vi "IO通讯.vi"(6 "baud rate (9600)":u32=9600 caption="波特率(9600)", 7 "VISA resource name":refnum<visa-resource-name> caption="VISA资源名称", 8 "错误输入（无错误）":errorcluster, 9 "操作":T1(ring), 10 "WRITE AND READ":string, 11 "WRITE":string) -> (0 "错误输出":errorcluster, 3 "READ":string)   [LabVIEW 2018, in "qingshan.lvlib"]
uses:
  qingshan/qingshan.lvlib
  <vilib>/Instr/_visa.llb/VISA Configure Serial Port (Instr).vi
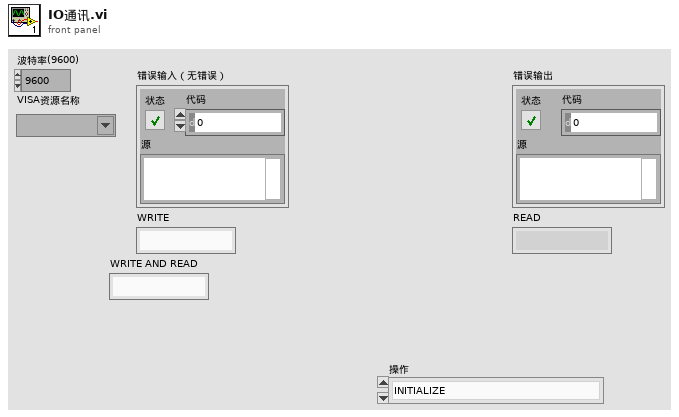
[diagram p1: front panel]
types:
  T1 = enum16{"INITIALIZE", "OPEN", "WRITE", "READ", "WRITE   AND  READ", "CLOSE", ""}
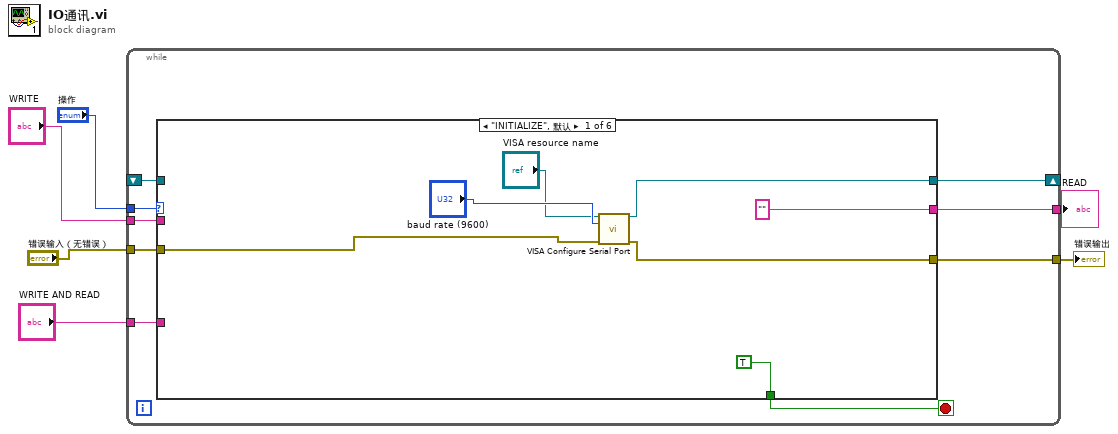
[diagram p0: block diagram]
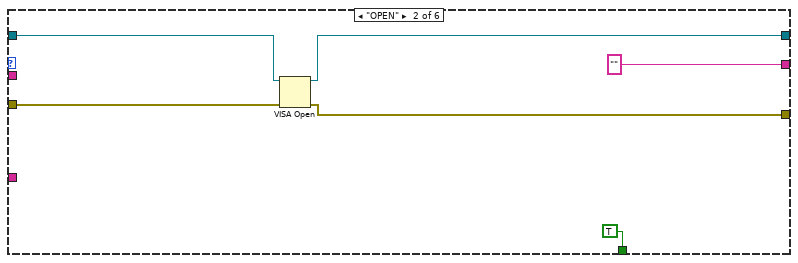
[diagram p2: hidden frame]
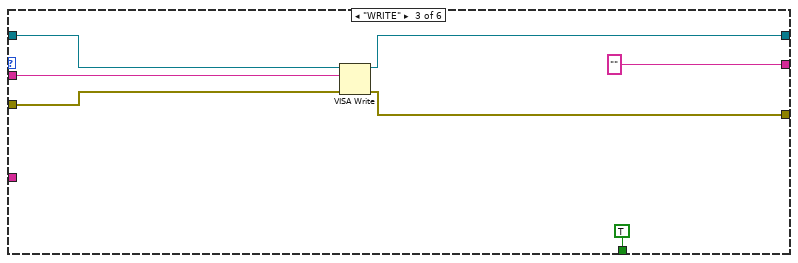
[diagram p3: hidden frame]
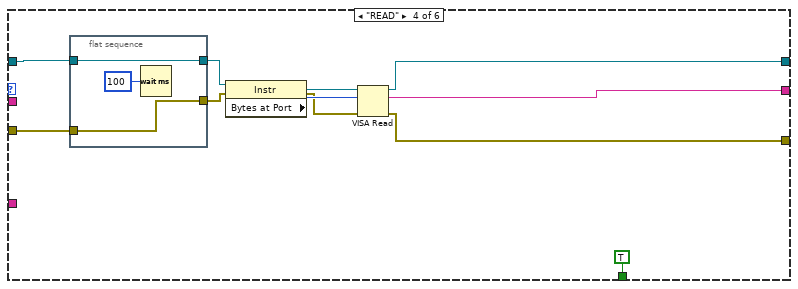
[diagram p4: hidden frame]
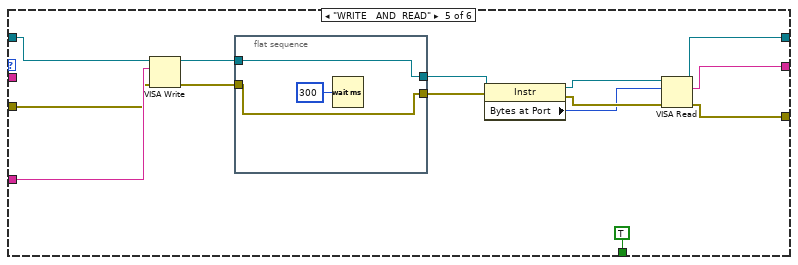
[diagram p5: hidden frame]
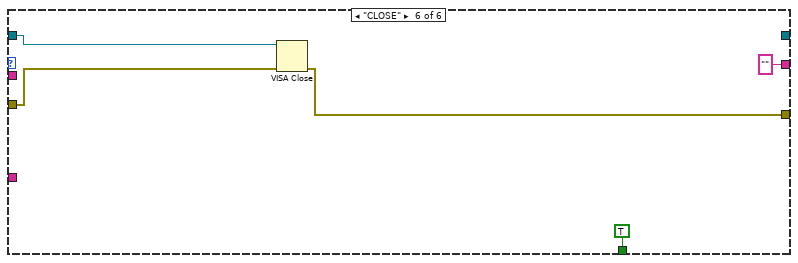
[diagram p6: hidden frame]
diagram:
  n1 = while {
    tunnel: "操作" -> [w15]
    shift-right: [w14] -> _
    shift-left: _ -> [w12]
    tunnel: "错误输入（无错误）" -> [w11]
    tunnel: [w10] -> w4
    tunnel: "WRITE" -> [w9]
    tunnel: [w8] -> w2
    tunnel: "WRITE AND READ" -> [w7]
    stop <- w13 stop-if-true
    n2 = case shown="\"INITIALIZE\", 默认" w15 {
      tunnel: [w22 w27 w34 w44 w52 _] -> w14
      tunnel: [TRUE TRUE TRUE TRUE TRUE TRUE] -> w13
      tunnel: w12 -> [_ w28 w35 w40 w62 w71]
      tunnel: w11 -> [w19 w25 w32 w38 w61 w70]
      tunnel: [w20 w24 w31 w43 w51 w69] -> w10
      tunnel: w9 -> [_ _ w33 _ _ _]
      tunnel: ["" ("read buffer") "" ("read buffer") "" ("read buffer") w42 w53 "" ("read buffer")] -> w8
      tunnel: w7 -> [_ _ _ _ w63 _]
      frame "INITIALIZE", Default {
        n3 = call-poly "VISA Configure Serial Port"("VISA resource name"="VISA resource name", "baud rate (9600)"="baud rate (9600)", "error in (no error)"=w19) -> ("VISA resource name out"=w22:refnum<visa-resource-name>, "error out"=w20:errorcluster)  [unwired: 11 in]
      }
      frame "OPEN" {
        n4 = VISA Open(error in (no error)=w25, VISA resource name=w28) -> (VISA resource name=w27:refnum<visa-resource-name>, error out=w24:errorcluster)  [unwired: 3 in]
      }
      frame "WRITE" {
        n5 = VISA Write(VISA resource name=w35, write buffer=w33, error in (no error)=w32) -> (VISA resource name out=w34:refnum<visa-resource-name>, error out=w31:errorcluster)  [unwired: 1 out]
      }
      frame "READ" {
        n6 = flat-sequence {
          tunnel: [w48] -> w41
          tunnel: w40 -> [w48]
          tunnel: [w47] -> w39
          tunnel: w38 -> [w47]
          frame #0 {
            n7 = Wait (ms)(milliseconds to wait=u32 100 ("等待时间（毫秒）")) -> ()  [unwired: 1 out]
          }
        }
        n8 = property class="Instr"(reference=w41, error in=w39) -> (reference out=w46:refnum<visa-resource-name>, error out=w37:errorcluster, "Bytes at Port"=w45:u32)
        n9 = VISA Read(VISA resource name=w46, byte count=w45, error in (no error)=w37) -> (VISA resource name out=w44:refnum<visa-resource-name>, read buffer=w42:string, error out=w43:errorcluster)  [unwired: 1 out]
      }
      frame "WRITE   AND  READ" {
        n10 = VISA Write(VISA resource name=w62, write buffer=w63, error in (no error)=w61) -> (VISA resource name out=w59:refnum<visa-resource-name>, error out=w57:errorcluster)  [unwired: 1 out]
        n11 = flat-sequence {
          tunnel: [w65] -> w60
          tunnel: w59 -> [w65]
          tunnel: [w64] -> w58
          tunnel: w57 -> [w64]
          frame #0 {
            n12 = Wait (ms)(milliseconds to wait=u32 300 ("等待时间（毫秒）")) -> ()  [unwired: 1 out]
          }
        }
        n13 = property class="Instr"(reference=w60, error in=w58) -> (reference out=w56:refnum<visa-resource-name>, error out=w55:errorcluster, "Bytes at Port"=w54:u32)
        n14 = VISA Read(VISA resource name=w56, byte count=w54, error in (no error)=w55) -> (VISA resource name out=w52:refnum<visa-resource-name>, read buffer=w53:string, error out=w51:errorcluster)  [unwired: 1 out]
      }
      frame "CLOSE" {
        n15 = VISA Close ("VISA关闭")(VISA resource name=w71, error in (no error)=w70) -> (error out=w69:errorcluster)
      }
    }
  }
  "错误输出" <- w4
  "READ" <- w2
